vi "Set Label Config.vi"(8 "error in (no error)":errorcluster, 11 "RT Data in":T1 {"Label Transfer Config"."Block Data Refs"."Data Reference" format="%.0x"; "Status Config"."HWOut Dur Ref" format="%.0x"; "Status Config"."HWIn Dur Ref" format="%.0x"; "Status Config"."Error Data Ref" format="%.0x"; "HWOutput Channels"."Labels Settings"."Label" format="%.0o"; "HWInput Channels"."Labels Settings"."Label" format="%.0o"}) -> (0 "error out":errorcluster, 3 "RT Data out":T1 {"Label Transfer Config"."Block Data Refs"."Data Reference" format="%.0x"; "Status Config"."HWOut Dur Ref" format="%.0x"; "Status Config"."HWIn Dur Ref" format="%.0x"; "Status Config"."Error Data Ref" format="%.0x"; "HWOutput Channels"."Labels Settings"."Label" format="%.0o"; "HWInput Channels"."Labels Settings"."Label" format="%.0o"})   [LabVIEW 2012, in "AIT 429 Engine.lvlib"]
uses:
  AIT 429 Engine.lvlib
  RT Controls/RT Data.ctl
  RT Controls/RT HW Channel.ctl
  RT Controls/RT Label Settings.ctl
  Shared/Controls and Global/Label.ctl
  Shared/Controls and Global/transferPeriod.ctl
  RT Controls/Driver Data.ctl
  RT Controls/RT Word Settings.ctl
  <vilib>/NI Veristand/Custom Device API/Block Data Reference.ctl
  <vilib>/NI Veristand/Custom Device API/Data Reference.ctl
  RT Controls/RT Param Setting.ctl
  Shared/Controls and Global/Start Bit.ctl
  Shared/Controls and Global/Number of Bits.ctl
  Shared/Controls and Global/TransferType.ctl
  RT Controls/Error Qs.ctl
  RT Controls/Status Channels Config.ctl
  RT Controls/FIFO.ctl
  RT Controls/Label Transfer Config.ctl
  SEA 9811 FPGA driver/RT/Typdefs/SEA9811_RT_data_cluster.ctl
  SEA 9811 FPGA driver/RT/Typdefs/FPGA ref.ctl
  SEA 9811 FPGA driver/RT/Typdefs/channel.ctl
  SEA 9811 FPGA driver/RT/Typdefs/received word.ctl
  <instrlib>/AIT 429/AIT 429.lvlib
  Shared/ARINC 429 Shared.lvlib
  <vilib>/NI Veristand/Custom Device API/Custom Device API.lvlib
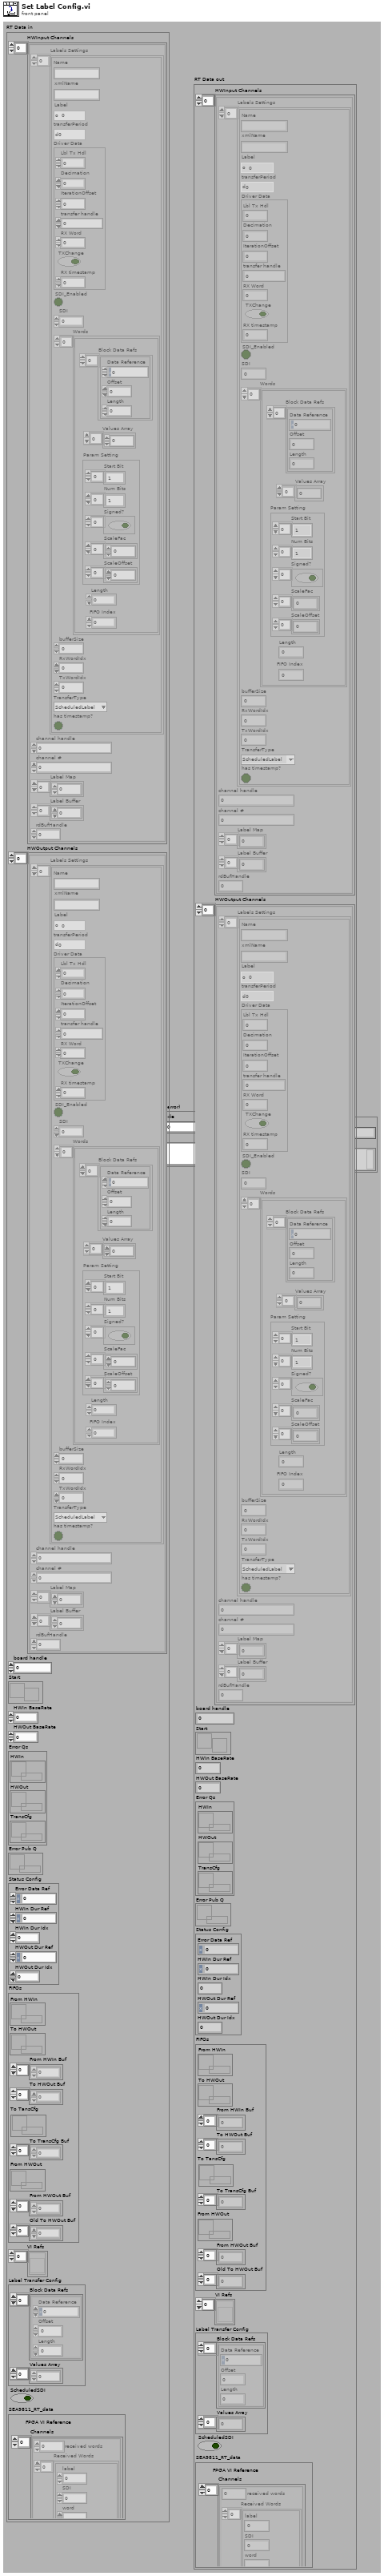
[diagram p1: front panel]
types:
  T1 = typedef "AIT 429 Engine.lvlib/RT Data.ctl" = cluster{"HWInput Channels":T2[], "HWOutput Channels":T2[], "board handle":u32, "Start":refnum<notifier>, "HWIn BaseRate":i64, "HWOut BaseRate":i64, "Error Qs":T14, "Error Pub Q":refnum<queue>, "Status Config":T15, "FIFOs":T16, "VI Refs":refnum<vi>[], "Label Transfer Config":T17, "ScheduledSDI":bool, "SEA9811_RT_data":T18}
  T2 = typedef "AIT 429 Engine.lvlib/RT HW Channel.ctl" = cluster{"Labels Settings":T3[], "channel handle":u32, "channel #":u16, "Label Map":i32[], "Label Buffer":u32[], "rdBufHandle":u32}
  T3 = typedef "AIT 429 Engine.lvlib/RT Label Settings.ctl" = cluster{"Name":string, "xmlName":string, "Label":T4, "transferPeriod":T5, "Driver Data":T6, "SDI_Enabled":bool, "SDI":u8, "Words":T7[], "bufferSize":u32, "RxWordIdx":i32, "TxWordIdx":i32, "TransferType":T13, "has timestamp?":bool}
  T4 = typedef "ARINC 429 Shared.lvlib/Label.ctl" = u8
  T5 = typedef "ARINC 429 Shared.lvlib/transferPeriod.ctl" = u32
  T6 = typedef "AIT 429 Engine.lvlib/Driver Data.ctl" = cluster{"Lbl Tx Hdl":u32, "Decimation":i32, "IterationOffset":i32, "transfer handle":u32, "RX Word":u32, "TXChange":bool, "RX timestamp":dbl}
  T7 = typedef "AIT 429 Engine.lvlib/RT Word Settings.ctl" = cluster{"Block Data Refs":T8[], "Values Array":dbl[], "Length":i32, "FIFO Index":i32, "Param Setting":T10}
  T8 = typedef "Custom Device API.lvlib/Block Data Reference.ctl" = cluster{"Data Reference":T9, "Offset":i32, "Length":i32}
  T9 = typedef "Custom Device API.lvlib/Data Reference.ctl" = i32
  T10 = typedef "AIT 429 Engine.lvlib/RT Param Setting.ctl" = cluster{"Start Bit":T11[], "Num Bits":T12[], "Signed?":bool[], "ScaleFac":dbl[], "ScaleOffset":dbl[]}
  T11 = typedef "ARINC 429 Shared.lvlib/Start Bit.ctl" = i32
  T12 = typedef "ARINC 429 Shared.lvlib/Number of Bits.ctl" = i32
  T13 = typedef "ARINC 429 Shared.lvlib/TransferType.ctl" = enum16{"ScheduledLabel", "Acyclic", "Block", "Strobe"}
  T14 = typedef "AIT 429 Engine.lvlib/Error Qs.ctl" = cluster{"HWIn":refnum<queue>, "HWOut":refnum<queue>, "TransCfg":refnum<queue>}
  T15 = typedef "AIT 429 Engine.lvlib/Status Channels Config.ctl" = cluster{"Error Data Ref":T9, "HWIn Dur Ref":T9, "HWIn Dur Idx":i32, "HWOut Dur Ref":T9, "HWOut Dur Idx":i32}
  T16 = typedef "AIT 429 Engine.lvlib/FIFO.ctl" = cluster{"From HWIn":refnum<k33>, "To HWOut":refnum<k33>, "From HWIn Buf":dbl[], "To HWOut Buf":dbl[], "To TansCfg":refnum<k33>, "To TransCfg Buf":dbl[], "From HWOut":refnum<k33>, "From HWOut Buf":dbl[], "Old To HWOut Buf":dbl[]}
  T17 = typedef "AIT 429 Engine.lvlib/Label Transfer Config.ctl" = cluster{"Block Data Refs":T8[], "Values Array":dbl[]}
  T18 = typedef "SEA9811_RT_data_cluster.ctl" = cluster{"FPGA VI Reference":T19, "Channels":T20[]}
  T19 = typedef "FPGA ref.ctl" = refnum<k20>
  T20 = typedef "channel.ctl" = cluster{"received words":u32, "Received Words":T21[]}
  T21 = typedef "received word.ctl" = cluster{"label":u8, "SDI":u8, "word":u32, "timestamp":dbl}
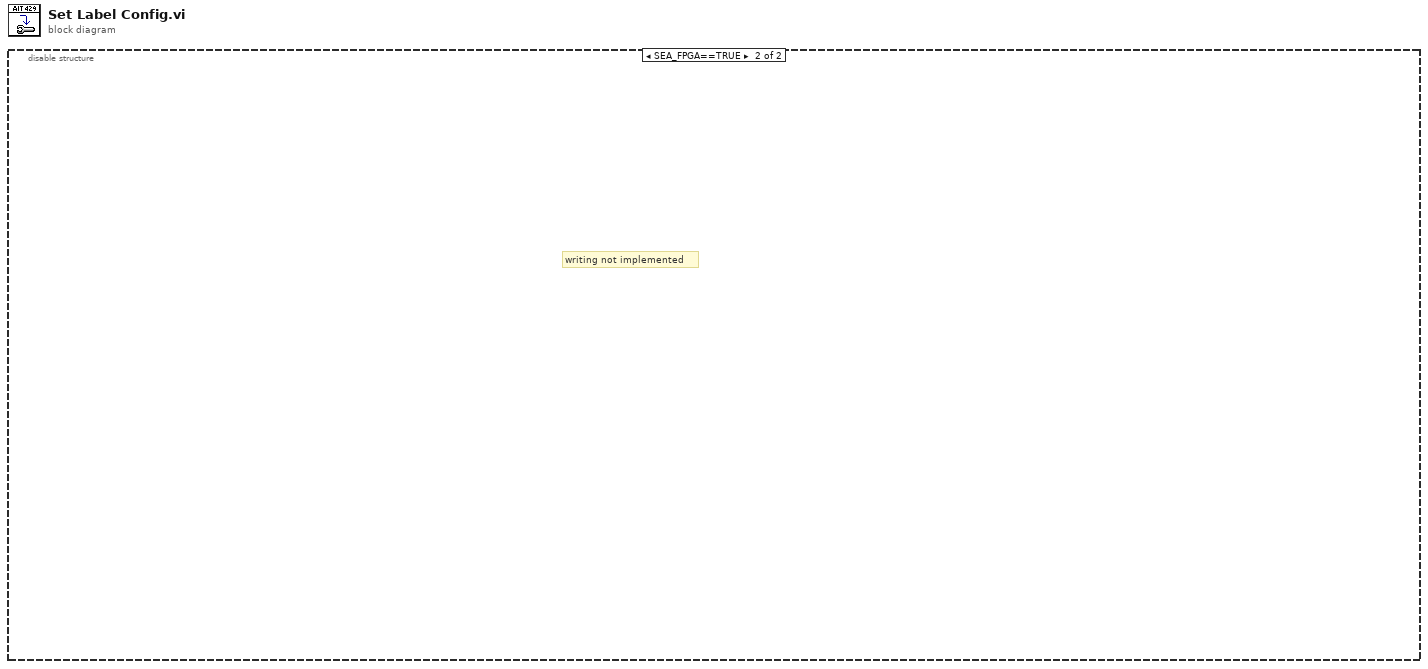
[diagram p0: block diagram]
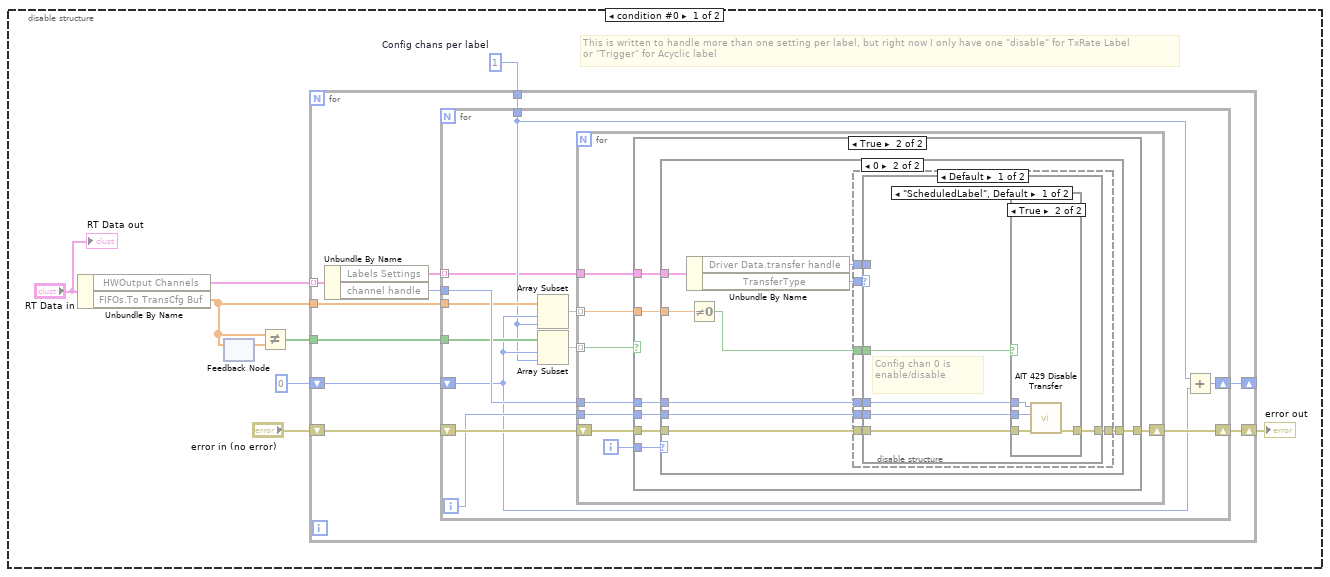
[diagram p2: hidden frame]
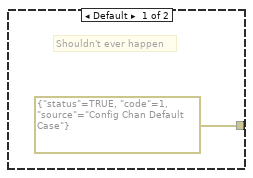
[diagram p4: hidden frame]
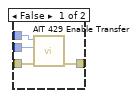
[diagram p5: hidden frame]
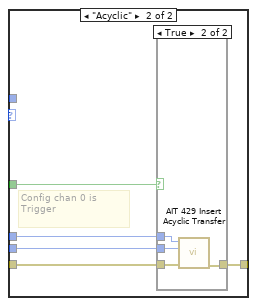
[diagram p6: hidden frame]
diagram:
  n1 = disable-structure shown="SEA_FPGA==TRUE" {
    frame condition #0 {
      w2 = 1  # Config chans per label
      # "This is written to handle more than one setting per label, but right now I only have one \"disable\" for TxRate Label \nor \"Trigger\" for Acyclic label"
      n2 = Unbundle By Name("RT Data in") -> ("HWOutput Channels"=w7:T2[], "FIFOs.To TransCfg Buf"=w1:dbl[])
      n3 = feedback #1() -> (w5:dbl[])  [unwired: 1 in]
      n4 = feedback-in #1(w1) -> ()
      n5 = Not Equal?(x=w1, y=w5) -> (x != y?=w4:bool[])
      n6 = for {
        shift-right: [w18] -> w8
        shift-left: "error in (no error)" -> [w19]
        tunnel: w7 -> [w17] mode=indexing
        shift-right: [w11] -> _
        shift-left: 0 ("index") -> [w13]
        tunnel: w4 -> [w14]
        tunnel: w2 -> [w12]
        tunnel: w1 -> [w10]
        n7 = Unbundle By Name(w17) -> ("Labels Settings"=w16:T3[], "channel handle"=w15:u32)
        n8 = for {
          tunnel: w16 -> [w20] mode=indexing
          tunnel: w15 -> [w29]
          shift-right: [w30] -> w18
          shift-left: w19 -> [w31]
          tunnel: w14 -> [w28]
          tunnel: w12 -> [w22]
          shift-right: [w26] -> w11
          shift-left: w13 -> [w23]
          tunnel: w10 -> [w24]
          i -> [w25]
          n9 = Array Subset(array=w24, index=w23, length=w22) -> (w21:dbl[])
          n10 = Array Subset(array=w28, index=w23, length=w22) -> (w27:bool[])
          n11 = for {
            tunnel: w29 -> [w37]
            tunnel: w27 -> [w35] mode=indexing
            tunnel: w25 -> [w36]
            shift-right: [w38] -> w30
            shift-left: w31 -> [w39]
            tunnel: w21 -> [w34] mode=indexing
            tunnel: w20 -> [w32]
            i -> [w33]
            n12 = case shown="True" w35 {
              tunnel: w39 -> [w40 w47]
              tunnel: [w40 w46] -> w38
              tunnel: w37 -> [_ w45]
              tunnel: w36 -> [_ w44]
              tunnel: w34 -> [_ w42]
              tunnel: w33 -> [_ w43]
              tunnel: w32 -> [_ w41]
              frame False {
              }
              frame True {
                n13 = case shown="0" w43 {
                  tunnel: w47 -> [_ w57]
                  tunnel: [errorcluster {"status"=TRUE, "code"=1, "source"="Config Chan Default Case"} ("error out") w56] -> w46
                  tunnel: w45 -> [_ w55]
                  tunnel: w44 -> [_ w54]
                  tunnel: w42 -> [_ w53]
                  tunnel: w41 -> [_ w51]
                  frame Default {
                    # "Shouldn't ever happen"
                  }
                  frame 0 {
                    n14 = Unbundle By Name(w51) -> ("Driver Data.transfer handle"=w49:u32, "TransferType"=w50:T13)
                    n15 = Not Equal To 0?(x=w53) -> (x != 0?=w52:bool)
                    n16 = disable-structure shown="Default" {
                      disable-tunnel: w57 -> [w64 w88]
                      disable-tunnel: [w63 w88] -> w56
                      disable-tunnel: w55 -> [w62 _]
                      disable-tunnel: w54 -> [w61 _]
                      disable-tunnel: w52 -> [w60 _]
                      disable-tunnel: w50 -> [w59 _]
                      disable-tunnel: w49 -> [w58 _]
                      frame condition #0 {
                        n17 = case shown="\"ScheduledLabel\", Default" w59 {
                          tunnel: w64 -> [w69 w82]
                          tunnel: [w68 w81] -> w63
                          tunnel: w62 -> [w67 w80]
                          tunnel: w61 -> [w66 w78]
                          tunnel: w60 -> [w65 w79]
                          tunnel: w58 -> [_ _]
                          frame "ScheduledLabel", Default {
                            # "Config chan 0 is enable/disable"
                            n18 = case shown="True" w65 {
                              tunnel: w69 -> [w72 w77]
                              tunnel: [w73 w76] -> w68
                              tunnel: w67 -> [w71 w75]
                              tunnel: w66 -> [w70 w74]
                              frame False {
                                n19 = call <instrlib>:"AIT 429 Enable Transfer.vi"("error in (no error)"=w72, "transfer handle in"=w70, "Tx channel handle in"=w71) -> ("error out"=w73:errorcluster)  [unwired: 7 in, 1 out]
                              }
                              frame True {
                                n20 = call <instrlib>:"AIT 429 Disable Transfer.vi"("error in"=w77, "transfer handle in"=w74, "Tx channel handle in"=w75) -> ("error out"=w76:errorcluster)  [unwired: 6 in, 2 out]
                              }
                            }
                          }
                          frame "Acyclic" {
                            # "Config chan 0 is \nTrigger"
                            n21 = case shown="True" w79 {
                              tunnel: w82 -> [w83 w87]
                              tunnel: [w83 w86] -> w81
                              tunnel: w80 -> [_ w85]
                              tunnel: w78 -> [_ w84]
                              frame False {
                              }
                              frame True {
                                n22 = call <instrlib>:"AIT 429 Insert Acyclic Transfer.vi"("error in (no error)"=w87, "acyclic handle"=w84, "channel handle"=w85) -> ("error out"=w86:errorcluster)  [unwired: 7 in, 1 out]
                              }
                            }
                          }
                        }
                      }
                      frame condition #1 (active) {
                      }
                    }
                  }
                }
              }
            }
          }
          n23 = Add(x=w22, y=w23) -> (x+y=w26:i32)
        }
      }
      "error out" <- w8
      "RT Data out" <- "RT Data in"
    }
    frame condition #1 (active) {
      # "writing not implemented"
    }
  }
